vi "Z Aux Execute.vi"(7 "uiResponseLength":u32, 8 "error in (no error)":errorcluster caption="错误输入（无错误）", 9 "psResponse":string, 10 "pszCommand":string, 11 "handle":u32) -> (0 "error out":errorcluster caption="错误输出", 1 "psResponse out":string, 2 "function return":i32, 3 "handle out":u32)   [LabVIEW 2015, in "zauxdll.lvlib"]
doc: "int32 __stdcall ZAux_Execute(ZMC_HANDLE handle, const char* pszCommand, char* psResponse, uint32 uiResponseLength);"
uses:
  zauxdll.lvlib
  zauxdll.dll
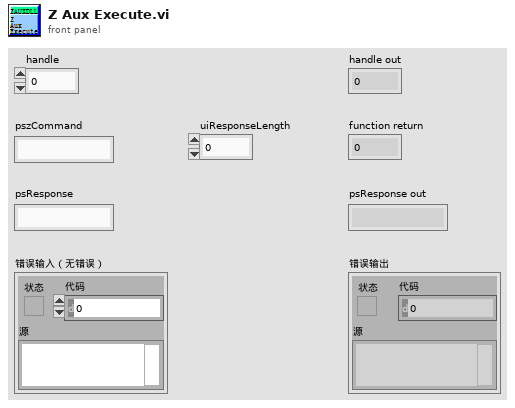
[diagram p1: front panel]
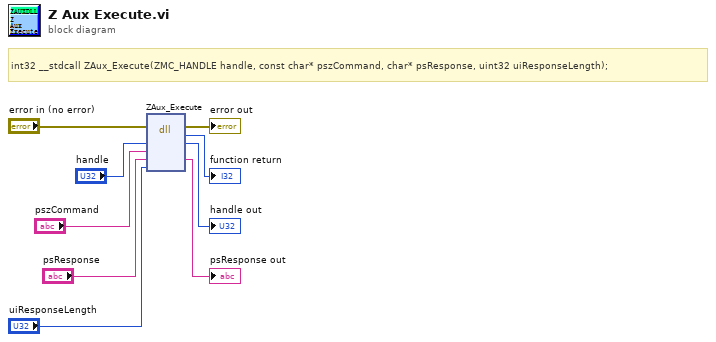
[diagram p0: block diagram]
diagram:
  # "int32 __stdcall ZAux_Execute(ZMC_HANDLE handle, const char* pszCommand, char* psResponse, uint32 uiResponseLength);"
  n1 = dll-call lib="C:/Users/VIC/Desktop/GOGORO_Oringnal - Panasonic/system/LLB/zmotion/zaux/zauxdll.*" fn="ZAux_Execute"(error in="error in (no error)", "handle"="handle", "pszCommand"="pszCommand", "psResponse"="psResponse", "uiResponseLength"="uiResponseLength") -> (error out=→"error out":errorcluster, →"function return":i32, "handle"=→"handle out":u32, "psResponse"=→"psResponse out":string)  [unwired: 4 in, 1 out]
